vi "TruncU16.vi"(5 "Decimal places":i8, 6 "Number":u16) -> (2 "Truncated number":u16)   [LabVIEW 2017, in "GPNumeric.lvlib"]
doc: "Truncates <B>Number</B> to a number of <B>Decimal places</B>.\n\nSet <B>Decimal places</B> to a negative number to truncate to nearest 10, nearest 100 and so on. E.g. to truncate 782 to the nearest hundred, you set <B>Decimal places</B> to -2 and the <B>Truncated number</B> will be 700.\n\nThis VI is inlined.\n\nSteen Schmidt\nGPower\n16/5 2014"
uses:
  GPNumeric.lvlib
panel:
  # "Copyright © 2014\nGPower\nSee enclosed license file for terms and conditions"
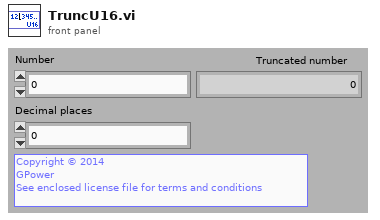
[diagram p1: front panel]
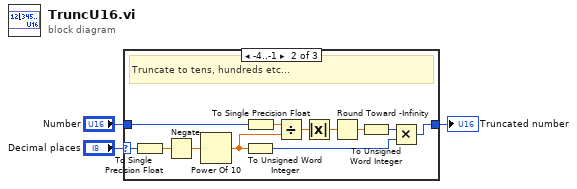
[diagram p0: block diagram]
diagram:
  n1 = case shown="-4..-1" "Decimal places" {
    selector: "Decimal places" -> [_ w12 _]
    tunnel: [_ w9 w16] -> w3
    tunnel: "Number" -> [_ w10 w16]
    frame ..-5 {
      # "Truncate above max value; Return zero."
    }
    frame -4..-1 {
      # "Truncate to tens, hundreds etc..."
      n2 = To Single Precision Float(number=w12) -> (single precision float=w11:sgl)
      n3 = Negate(x=w11) -> (-x=w15:sgl)
      n4 = Power Of 10(x=w15) -> (10^x=w8:sgl)
      n5 = To Unsigned Word Integer(number=w8) -> (unsigned 16bit integer=w14:u16)
      n6 = To Single Precision Float(number=w10) -> (single precision float=w6:sgl)
      n7 = Divide(x=w6, y=w8) -> (x/y=w5:sgl)
      n8 = Absolute Value(x=w5) -> (abs(x)=w7:sgl)
      n9 = Round Toward -Infinity(1:w7) -> (0:w4:sgl)
      n10 = To Unsigned Word Integer(number=w4) -> (unsigned 16bit integer=w13:u16)
      n11 = Multiply(x=w13, y=w14) -> (x*y=w9:u16)
    }
    frame 0.. {
      # "Truncate to n decimal places; return integer unchanged."
    }
  }
  "Truncated number" <- w3
